vi "GPS-Time.vi"(2 "错误In":errorcluster, 3 "响应":string) -> (0 "错误Out":errorcluster, 1 "时间":T1)   [LabVIEW 2015]
panel:
  out "数组":u16[](array[numeric])
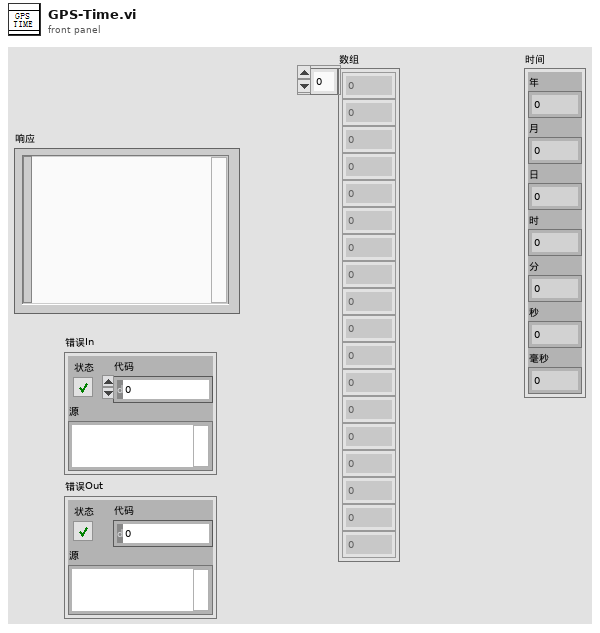
[diagram p1: front panel]
types:
  T1 = cluster{"年":u16, "月":u16, "日":u16, "时":u16, "分":u16, "秒":u16, "毫秒":u16}
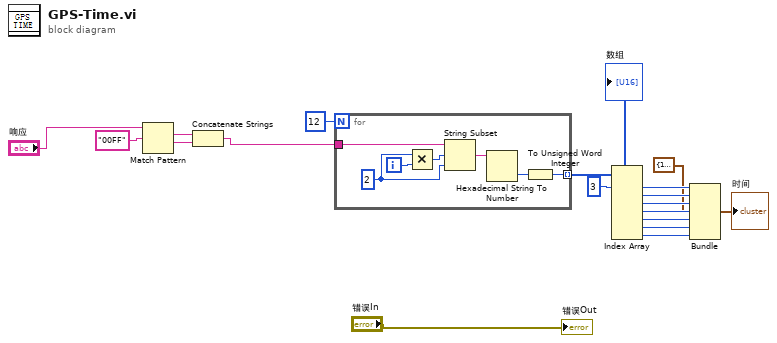
[diagram p0: block diagram]
diagram:
  n1 = Match Pattern(string="响应", regular expression="00FF" ("正则表达式")) -> (match substring=w5:string, after substring=w4:string)  [unwired: 1 in, 2 out]
  n2 = Concatenate Strings(w5, w4) -> (w3:string)
  n3 = for {
    N: 12 -> [_]
    tunnel: w3 -> [w25]
    tunnel: [w21] -> w18 mode=indexing
    i -> [w22]
    w23 = 2 ("偏移量(0)")
    n4 = Multiply(x=w23, y=w22) -> (x*y=w24:i32)
    n5 = String Subset(string=w25, offset (0)=w24, length (rest)=w23) -> (substring=w20:string)
    n6 = Hexadecimal String To Number(string=w20) -> (number=w19:u32)  [unwired: 2 in, 1 out]
    n7 = To Unsigned Word Integer(number=w19) -> (unsigned 16bit integer=w21:u16)
  }
  "数组" <- w18
  n8 = Index Array(array=w18, index #1=3 ("索引")) -> (element #1=w16:u16, element #2=w15:u16, element #3=w14:u16, element #4=w13:u16, element #5=w12:u16, element #6=w11:u16, element #7=w10:u16)  [unwired: 6 in]
  n9 = Bundle(cluster=T1 {"年"=18, "月"=11, "日"=5, "时"=11, "分"=11, "秒"=33, "毫秒"=217} ("簇"), "年"=w16, "月"=w15, "日"=w14, "时"=w13, "分"=w12, "秒"=w11, "毫秒"=w10) -> (→"时间":T1)
  "错误Out" <- "错误In"
